vi "MRC Smart IO Set Led Buffer.vi"(8 "error in (no error)":errorcluster, 10 "bufferLength":i32, 11 "buffer Data":u8[](array[numeric])) -> (0 "error out":errorcluster)   [LabVIEW 2026, in "MrcLib.lvlib"]
doc: "MRC_Status MRC_CALLCONV MRC_SmartIO_SetLedBuffer(uint8_t* ledBuffer, int32_t bufferLength);"
uses:
  MrcLib.lvlib
  MrcLib.so
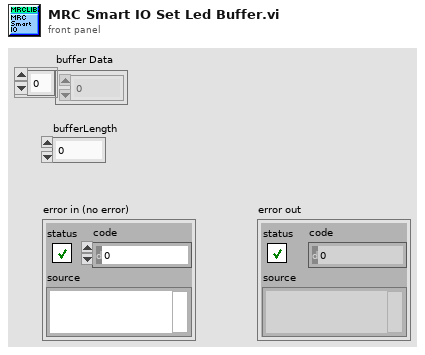
[diagram p1: front panel]
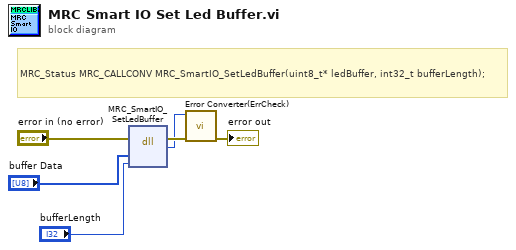
[diagram p0: block diagram]
diagram:
  # "MRC_Status MRC_CALLCONV MRC_SmartIO_SetLedBuffer(uint8_t* ledBuffer, int32_t bufferLength);"
  n1 = dll-call lib="MrcLib.*" fn="MRC_SmartIO_SetLedBuffer"(error in="error in (no error)", "ledBuffer"="buffer Data", "bufferLength"="bufferLength") -> (error out=w3:errorcluster, "return type"=w1:i32)  [unwired: 4 in, 1 out]
  n2 = call "Error Converter(ErrCheck).vi"("error in (no error)"=w3, "status"=w1) -> ("error out"=→"error out":errorcluster)  [unwired: 9 in]
